vi "uA__daq_Get_diana_uA_Vbat_for_reading.vi"(8 "error in (no error)":errorcluster, 10 "Coef":dbl, 11 "Refnum in":refnum<k21>) -> (0 "error out":errorcluster, 1 "Vbat":dbl, 2 "UA":waveform(dbl)(graph), 3 "uA Current":dbl, 4 "mA_offsect":dbl, 5 "task out":refnum<k21>)   [LabVIEW 2015]
uses:
  <vilib>/DAQmx/read.llb/DAQmx Read (Analog 1D Wfm NChan NSamp).vi
  <vilib>/DAQmx/miscellaneous.llb/DAQmx Fill In Error Info.vi
panel:
  out "uA_bank1":dbl
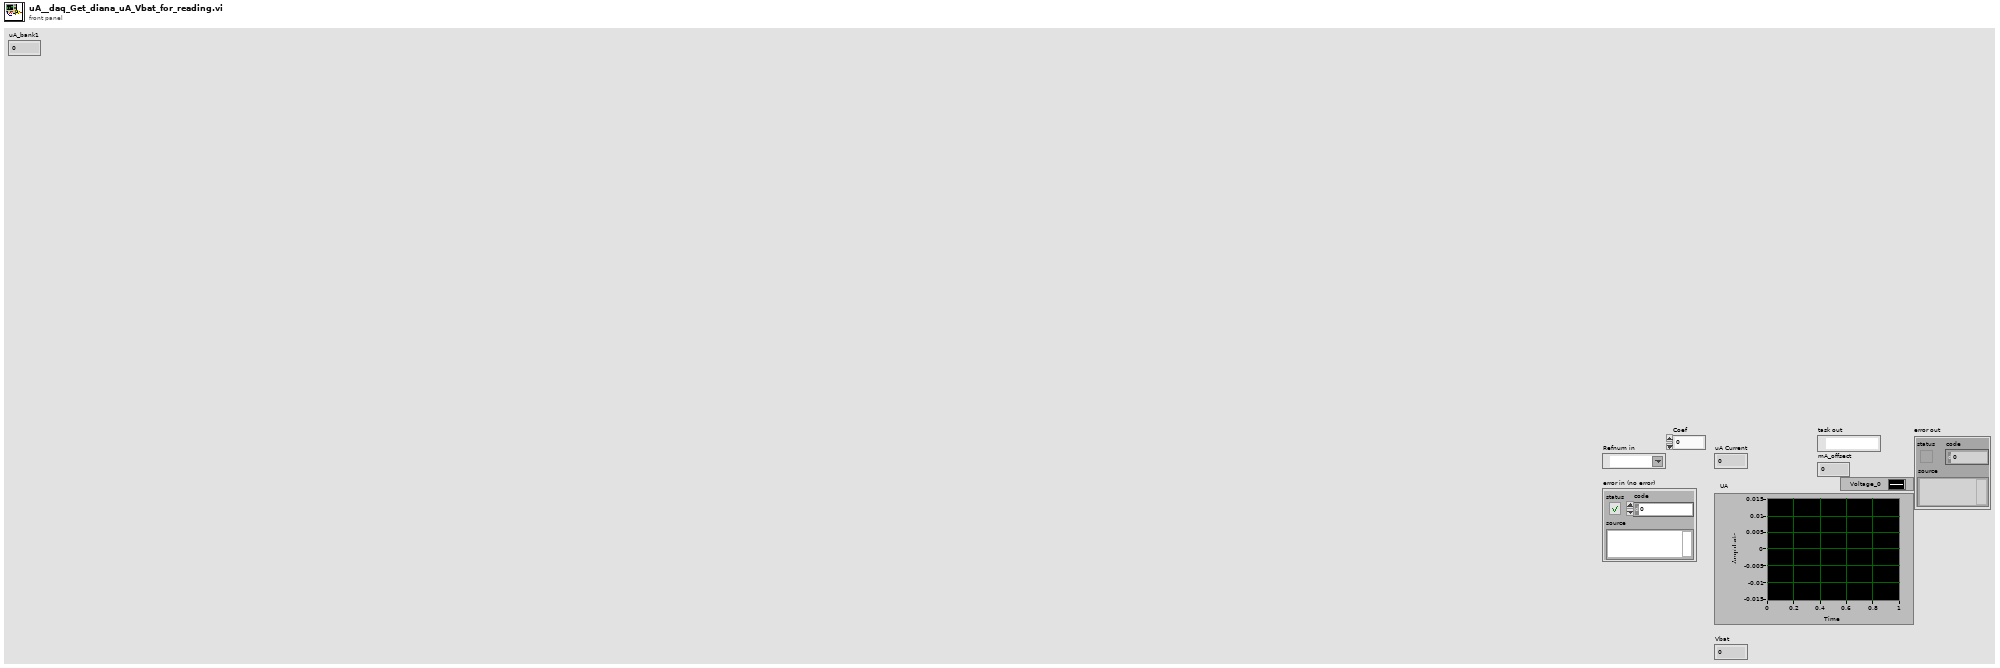
[diagram p1: front panel]
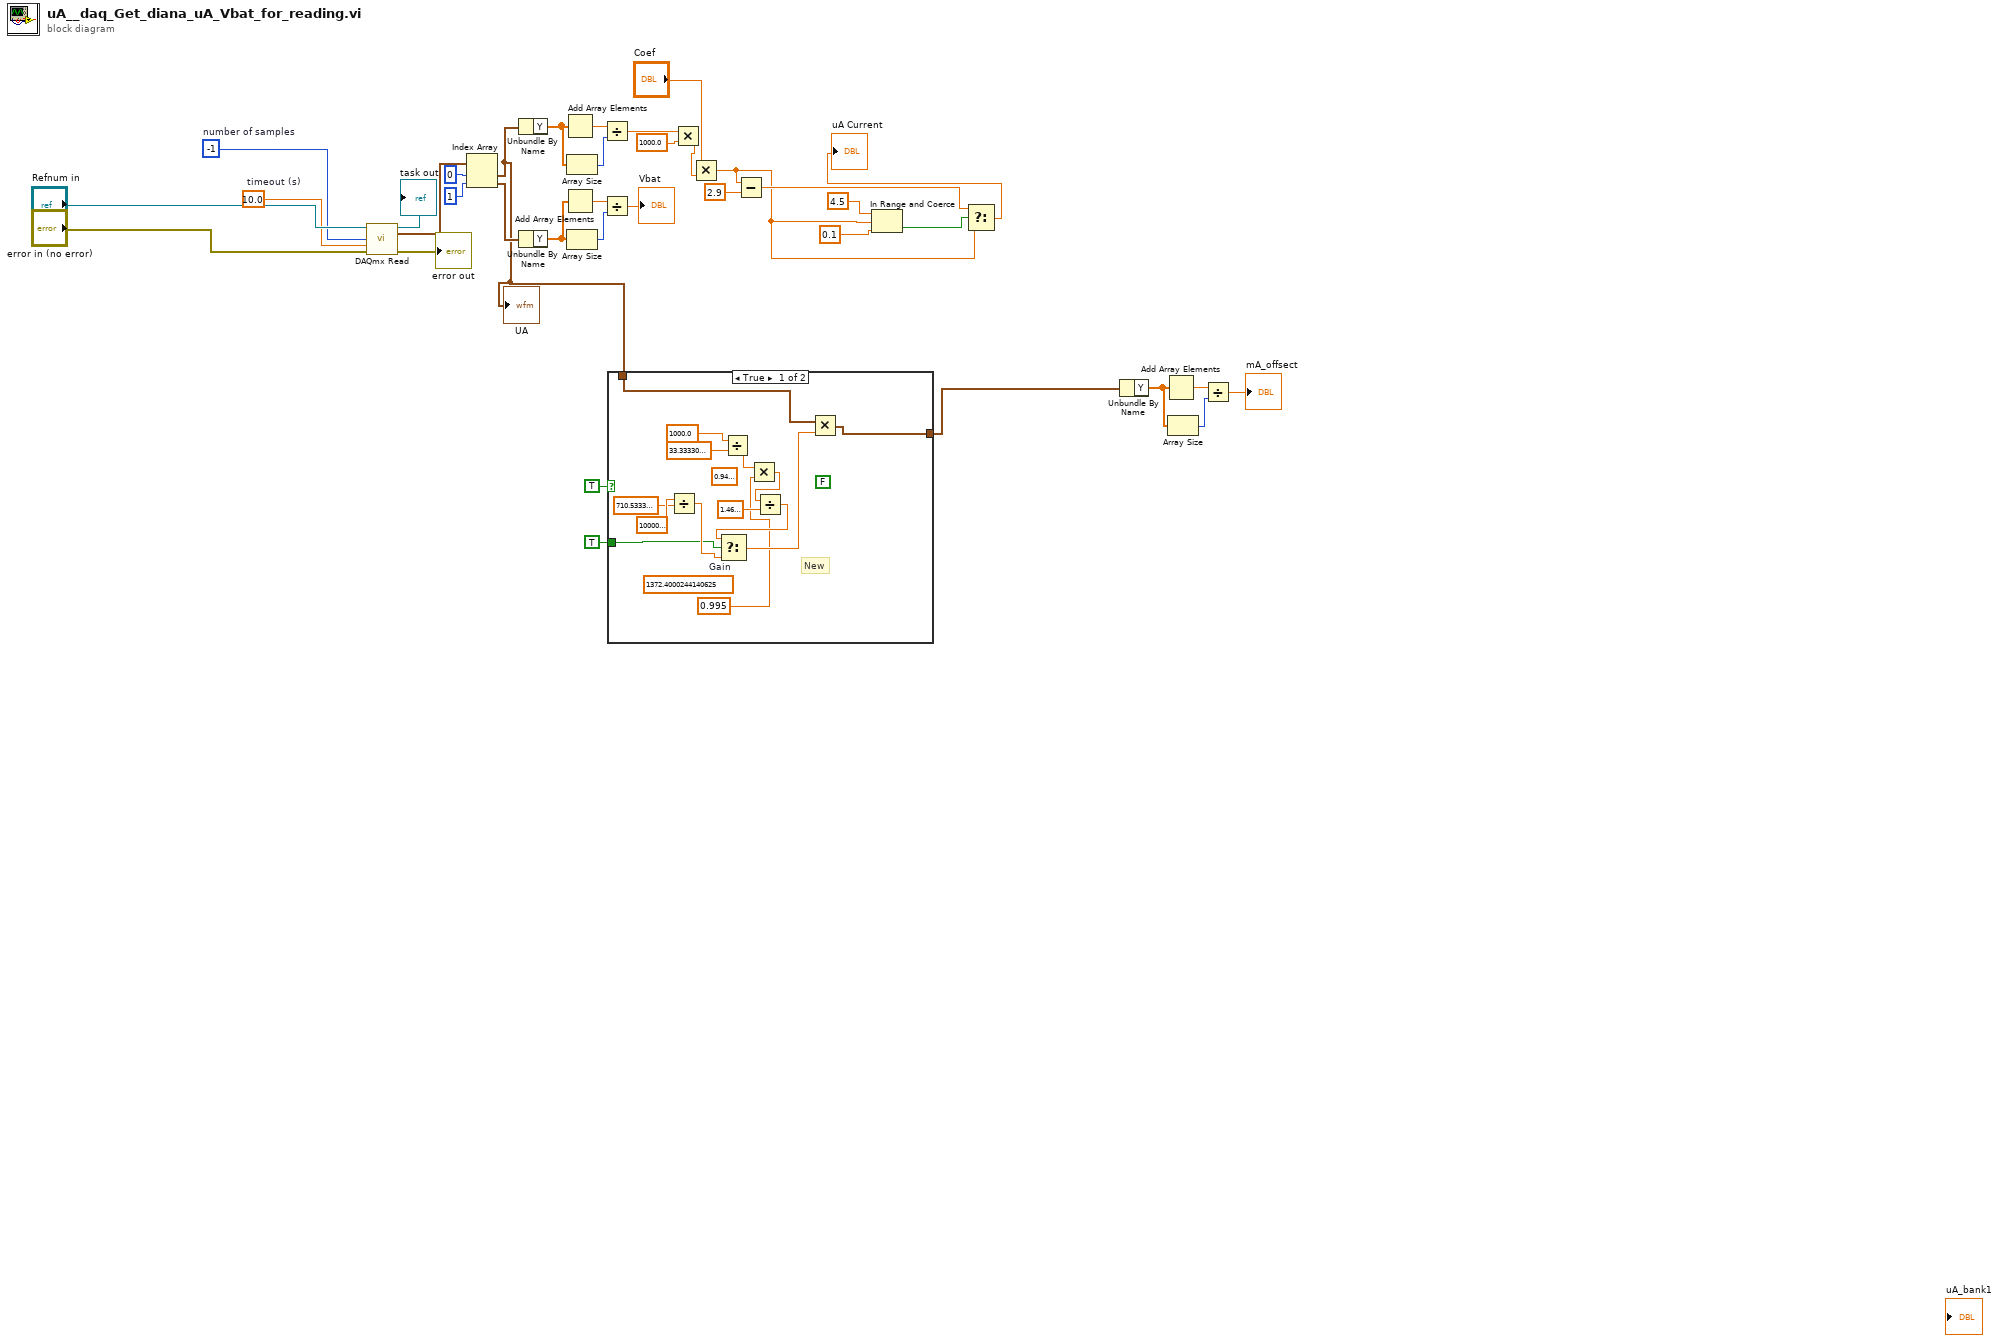
[diagram p0: block diagram]
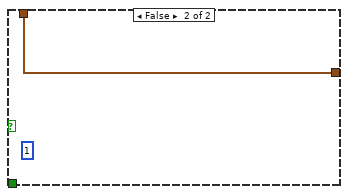
[diagram p2: hidden frame]
diagram:
  w22 = 10.0  # timeout (s)
  w21 = -1  # number of samples
  n1 = call-poly <vilib>:"DAQmx Read.vi"("task/channels in"="Refnum in", "number of samples per channel"=w21, "timeout"=w22, "error in"="error in (no error)") -> ("task out"=→"task out":refnum<k21>, "data"=w25:waveform(dbl)[], "error out"=→"error out":errorcluster)  [unwired: 9 in]
  n2 = Index Array(array=w25, index #1=0 ("index"), index #2=1 ("index")) -> (element #1=w6:waveform(dbl), element #2=w17:waveform(dbl))
  "UA" <- w6
  n3 = Unbundle By Name(w6) -> ("Y"=w29:dbl[])
  n4 = Unbundle By Name(w17) -> ("Y"=w34:dbl[])
  n5 = Add Array Elements(numeric array=w29) -> (sum=w28:dbl)
  n6 = Add Array Elements(numeric array=w34) -> (sum=w35:dbl)
  n7 = Array Size(array=w29) -> (size(s)=w30:i32)
  n8 = Array Size(array=w34) -> (size(s)=w33:i32)
  n9 = Divide(x=w28, y=w30) -> (x/y=w31:dbl)
  n10 = Divide(x=w35, y=w33) -> (x/y=→"Vbat":dbl)
  n11 = case shown="True" TRUE {
    tunnel: [w42 w51] -> w2
    tunnel: TRUE ("Value") -> [w43 _]
    tunnel: w6 -> [w37 w51]
    frame True {
      (unwired) FALSE
      (unwired) sgl 0.95 ("y")
      (unwired) sgl 1372.4  # Gain
      # "New"
      n12 = Divide(x=sgl 1000000.0, y=sgl 710.5333) -> (x/y=w46:sgl)
      n13 = Divide(x=sgl 1000.0 ("y"), y=sgl 33.3333) -> (x/y=w45:sgl)
      n14 = Multiply(x=w45, y=0.995 ("Numeric")) -> (x*y=w41:dbl)
      n15 = Divide(x=w41, y=sgl 1.46) -> (x/y=w40:dbl)
      n16 = Select(t=w40, s=w43, f=w46) -> (s? t:f=w48:dbl)
      n17 = Multiply(x=w37, y=w48) -> (x*y=w42:waveform(dbl))
    }
    frame False {
      (unwired) u16 1 ("Index")
    }
  }
  n18 = Multiply(x=w31, y=1000.0) -> (x*y=w19:dbl)
  n19 = Multiply(x="Coef", y=w19) -> (x*y=w12:dbl)
  n20 = Subtract(x=w12, y=2.9) -> (x-y=w14:dbl)
  n21 = In Range and Coerce(upper limit=4.5, x=w12, lower limit=0.1 ("y")) -> (In Range?=w15:bool)  [unwired: 1 out]
  n22 = Select(t=w14, s=w15, f=w12) -> (s? t:f=→"uA Current":dbl)
  n23 = Unbundle By Name(w2) -> ("Y"=w4:dbl[])
  n24 = Add Array Elements(numeric array=w4) -> (sum=w3:dbl)
  n25 = Array Size(array=w4) -> (size(s)=w5:i32)
  n26 = Divide(x=w3, y=w5) -> (x/y=→"mA_offsect":dbl)
